vi "RandomNumberGeneratorv2.vi"(11 "In Play Array":i32[](array[numeric])=[1, 1, 1, 1, 1, 1, 1, 1, 1, 1, 1, 1, 1, 1, 1, 1, 1, 1]) -> (3 "Index":u8)   [LabVIEW 2018]
panel:
  out "Random Number":u8
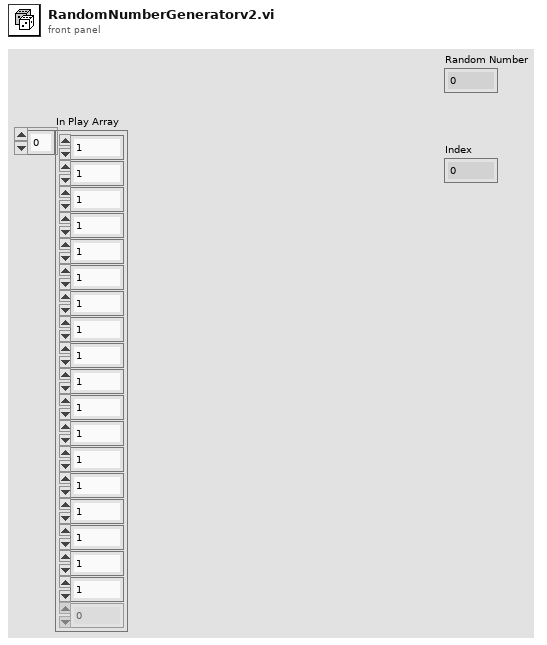
[diagram p1: front panel]
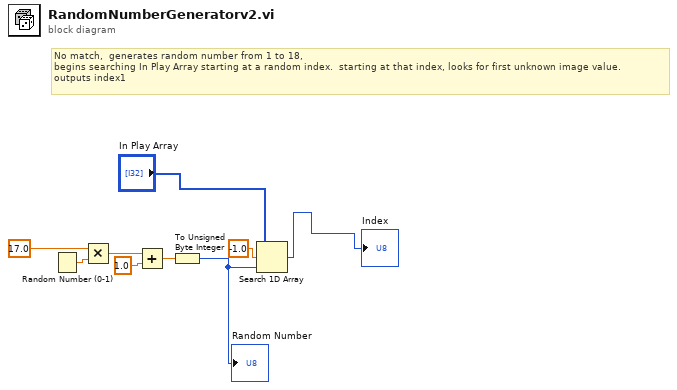
[diagram p0: block diagram]
diagram:
  # "No match,  generates random number from 1 to 18, \nbegins searching In Play Array starting at a random index.  starting at that index, looks for first unknown image value.\noutputs index1"
  n1 = Random Number (0-1)() -> (number: 0 to 1=w8:dbl)
  n2 = Multiply(x=17.0, y=w8) -> (x*y=w6:dbl)
  n3 = Add(x=w6, y=1.0) -> (x+y=w5:dbl)
  n4 = To Unsigned Byte Integer(number=w5) -> (unsigned 8bit integer=w4:u8)
  "Random Number" <- w4
  n5 = Search 1D Array(1D array="In Play Array", element=-1.0, start index (0)=w4) -> (index of element=→"Index":i32)
